vi "Load Sweep Table.vi"(7 "Axis (0: swpInner)":i32(ring) items=["swpInner", "swpOuter"], 8 "error in (no error)":errorcluster, 9 "Column Index (0)":i32, 10 "Table File Name (\"MyFile.txt\")":string="\"MyFile.txt\"", 11 "VISA resource name":refnum<visa-resource-name>) -> (0 "error out":errorcluster, 3 "VISA resource name out":refnum<visa-resource-name>)   [LabVIEW 2014, in "Stanford Research SR1.lvlib"]
doc: "Loads Sweep Table data fromthe specified column of the named file."
uses:
  Stanford Research SR1.lvlib
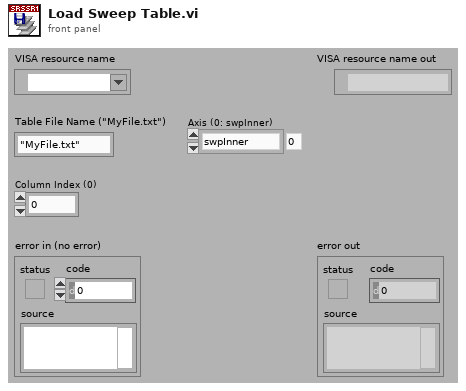
[diagram p1: front panel]
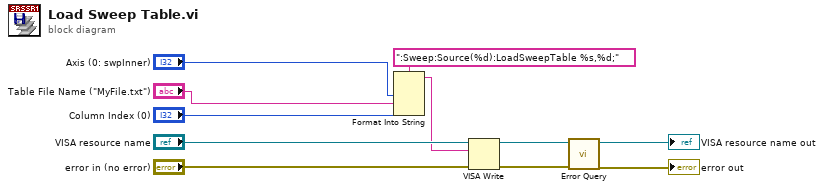
[diagram p0: block diagram]
diagram:
  n1 = Format Into String(format string=":Sweep:Source(%d):LoadSweepTable %s,%d;", "Axis (0: swpInner)", "Table File Name (\"MyFile.txt\")", "Column Index (0)") -> (resulting string=w1:string)  [unwired: 2 in, 1 out]
  n2 = VISA Write(VISA resource name="VISA resource name", write buffer=w1, error in (no error)="error in (no error)") -> (VISA resource name out=w8:refnum<visa-resource-name>, error out=w7:errorcluster)  [unwired: 1 out]
  n3 = call "Error Query.vi"("error in (no error)"=w7, "VISA resource name"=w8) -> ("error out"=→"error out":errorcluster, "VISA resource name out"=→"VISA resource name out":refnum<visa-resource-name>)  [unwired: 6 in, 2 out]
